vi "tiempo ejecucion calculo.vi"() -> ()   [LabVIEW 2016]
panel:
  out "time to match":dbl
  out "current number":dbl
  out "Number of iterations":dbl
  in  "NUmber to match":dbl
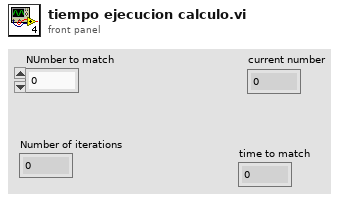
[diagram p1: front panel]
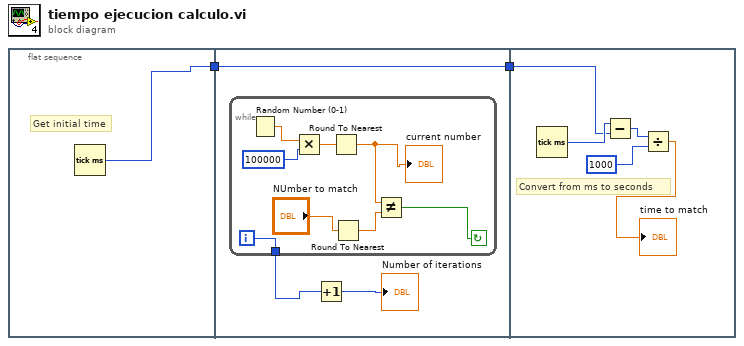
[diagram p0: block diagram]
diagram:
  n1 = flat-sequence {
    tunnel: [w3] -> w1
    tunnel: [w4] -> w2
    tunnel: w1 -> [w4]
    tunnel: w2 -> [w18]
    frame #0 {
      # "Get initial time"
      n2 = Tick Count (ms)() -> (millisecond timer value=w3:u32)
    }
    frame #1 {
      n3 = while {
        tunnel: [w7] -> w6
        i -> [w7]
        stop <- w8 continue-if-true
        n4 = Random Number (0-1)() -> (number: 0 to 1=w14:dbl)
        n5 = Multiply(x=w14, y=100000) -> (x*y=w12:dbl)
        n6 = Round To Nearest(number=w12) -> (nearest integer value=w9:dbl)
        "current number" <- w9
        n7 = Round To Nearest(number="NUmber to match") -> (nearest integer value=w10:dbl)
        n8 = Not Equal?(x=w9, y=w10) -> (x != y?=w8:bool)
      }
      n9 = Increment(x=w6) -> (x+1=→"Number of iterations":i32)
    }
    frame #2 {
      # "Convert from ms to seconds"
      n10 = Tick Count (ms)() -> (millisecond timer value=w19:u32)
      n11 = Subtract(x=w19, y=w18) -> (x-y=w17:u32)
      n12 = Divide(x=w17, y=1000) -> (x/y=→"time to match":dbl)
    }
  }
